vi "Save_Array_of_Products_to_File.vi"(10 "Path":path, 11 "array of #typedef Products":T1[](array[typedef])) -> ()   [LabVIEW 2020]
doc: "This VI saves <b>array of #typedef Products</b> into the text file stored in location gived by a <b>path</b>. Program seperates every element of cluster by comma."
uses:
  #typedef_Product.ctl
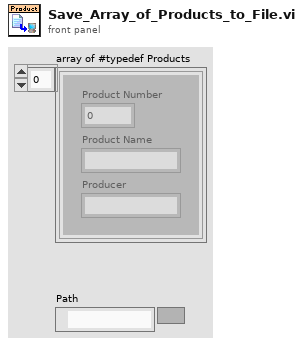
[diagram p1: front panel]
types:
  T1 = typedef "#typedef_Product.ctl" = cluster{"Product Number":i32, "Product Name":string, "Producer":string}
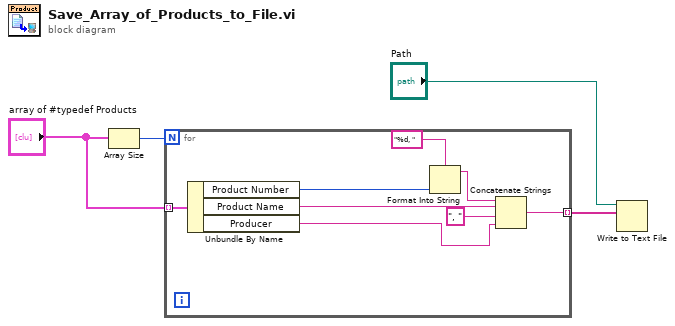
[diagram p0: block diagram]
diagram:
  n1 = Array Size(array="array of #typedef Products") -> (size(s)=w1:i32)
  n2 = for {
    N: w1 -> [_]
    tunnel: "array of #typedef Products" -> [w12] mode=indexing
    tunnel: [w5] -> w3 mode=indexing
    n3 = Unbundle By Name(w12) -> ("Product Number"=w11:i32, "Product Name"=w8:string, "Producer"=w6:string)
    n4 = Format Into String(format string="%d, ", w11) -> (resulting string=w9:string)  [unwired: 2 in, 1 out]
    n5 = Concatenate Strings(w9, w8, ", " ("string"), w6) -> (w5:string)
  }
  n6 = Write to Text File(file (use dialog)="Path", text=w3) -> ()  [unwired: 2 in, 3 out]
